vi "start.vi"(8 "error in (no error)":errorcluster, 11 "WriteSignalsGenericPlugin in":refnum<class "SignalWriterDL101123SoundCard.lvclass">) -> (0 "error out":errorcluster, 3 "WriteSignalsGenericPlugin out":refnum<class "SignalWriterDL101123SoundCard.lvclass">)   [LabVIEW 2010, in "SignalWriterDL101123SoundCard.lvclass"]
uses:
  SignalWriterDL101123SoundCard.lvclass
  SignalWriterDL101123SoundCard.lvclass/SignalWriterDL101123SoundCard.ctl
  <vilib>/sound2/lvsound2.llb/Sound Output Write (DBL Single).vi
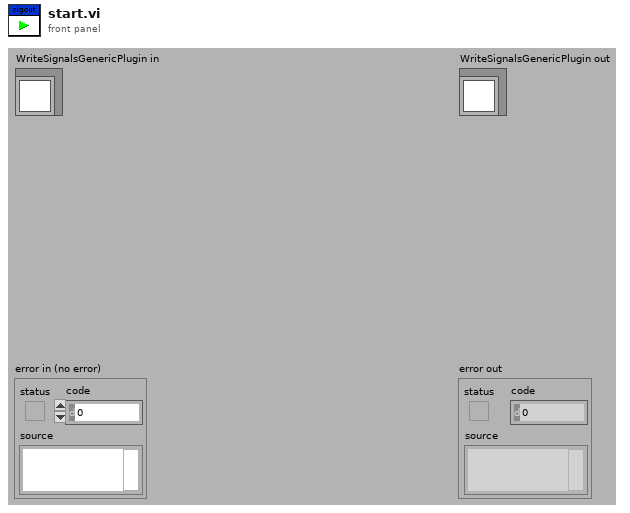
[diagram p1: front panel]
types:
  T1 = typedef "Sound Output Task ID.ctl" = u32
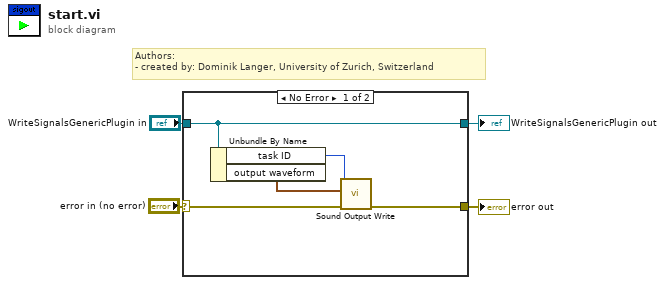
[diagram p0: block diagram]
diagram:
  # "Authors: \n- created by: Dominik Langer, University of Zurich, Switzerland"
  n1 = case shown="No Error" "error in (no error)" {
    selector: "error in (no error)" -> [w8 w11]
    tunnel: "WriteSignalsGenericPlugin in" -> [w9 w10]
    tunnel: [w7 w11] -> w2
    tunnel: [w9 w10] -> w1
    frame No Error {
      n2 = Unbundle By Name(w9) -> ("task ID"=w6:T1, "output waveform"=w5:waveform(dbl))
      n3 = call-poly <vilib>:"Sound Output Write.vi"("error in (no error)"=w8, "data"=w5, "task ID"=w6) -> ("error out"=w7:errorcluster)  [unwired: 7 in, 1 out]
    }
    frame Error {
    }
  }
  "error out" <- w2
  "WriteSignalsGenericPlugin out" <- w1
